vi "cRIO Main.vi"() -> ()   [LabVIEW 2015]
doc: "This application launches and executes the Tag Bus Data framework configuration for the specified target alias. This is a simple example of the framework API functions, but may also be a suitable starting point for a Host UI or Thick Client that is running a local version of the framework."
uses:
  <vilib>/NI/Module Execution Interface/Engine Runtime/Execution States.ctl
  <vilib>/NI/Module Execution Interface/Engine Runtime/Fault.ctl
  <vilib>/NI/Tag Bus Module Framework/runtime/error classification.ctl
  <vilib>/Utility/RT CPU Load.ctl
  <vilib>/NI/Current Value Table/DataTypes/Double_Read.vi
  <vilib>/NI/Current Value Table/DataTypes/U64_Read.vi
  <vilib>/NI/Current Value Table/DataTypes/U32_Read.vi
  <vilib>/NI/Current Value Table/DataTypes/Boolean_Read.vi
  <vilib>/NI/Current Value Table/Type to Enum.vi
  <vilib>/NI/Current Value Table/DataTypes/Double_Type To Enum.vi
  <vilib>/NI/Current Value Table/DataTypes/U64_Type To Enum.vi
  <vilib>/NI/Current Value Table/DataTypes/U32_Type To Enum.vi
  <vilib>/NI/Current Value Table/DataTypes/Boolean_Type To Enum.vi
  <vilib>/NI/Current Value Table/FGVs/CVT Globals.vi
  <vilib>/NI/Current Value Table/FGVs/Tag Memory.vi
  <vilib>/NI/Current Value Table/Memory Block.vi
  <vilib>/NI/Current Value Table/DataTypes/Boolean_Memory Block.vi
  <vilib>/NI/Current Value Table/DataTypes/U32_Memory Block.vi
  <vilib>/NI/Current Value Table/DataTypes/U64_Memory Block.vi
  <vilib>/NI/Current Value Table/DataTypes/Double_Memory Block.vi
  <vilib>/NI/Module Execution Interface/Engine Runtime/Engine Runtime Interface.lvclass
  <vilib>/NI/DCAF/Tag Editor Core/Framework Configuration Classes/target runtime/PL_Target Runtime.lvclass
  <vilib>/NI/Tag Bus Module Framework/runtime/TBM module execution interface.lvclass
  <vilib>/NI/Current Value Table/Current Value Table.lvlib
  <vilib>/NI_Real-Time Target Support.lvlib
panel:
  out "CPU loads":T1[](array[typedef]) {"ISR (%)" format="%#.2f"; "Idle (%)" format="%#.2f"; "Background (%)" format="%#.2f"; "Normal (%)" format="%#.2f"; "Above Normal (%)" format="%#.2f"; "High (%)" format="%#.2g"; "Timed Structures (%)" format="%#.2g"; "Time Critical (%)" format="%#.2g"; "Total (%)" format="%#.2g"}
  out "Time Structures":dbl
  out "Total":dbl
  in  "stop 2":bool
  out "error out 2":errorcluster
  out "Exec Time":u64
  out "Iterate DT":u64
  out "Late Count":u32
  out "Late":bool
  out "error out":errorcluster
  out "Duration Outputs":dbl
  out "Duration Process":dbl
  out "Duration Inputs":dbl
  out "Iter Start Time":dbl
  in  "configuration file path":path=path "/home/lvuser/benchmark_scan_IO_2x9205.pcfg"
  in  "target alias":string="dcaf_9068"
  out "engine status":T5(array[cluster])
  in  "stop":bool
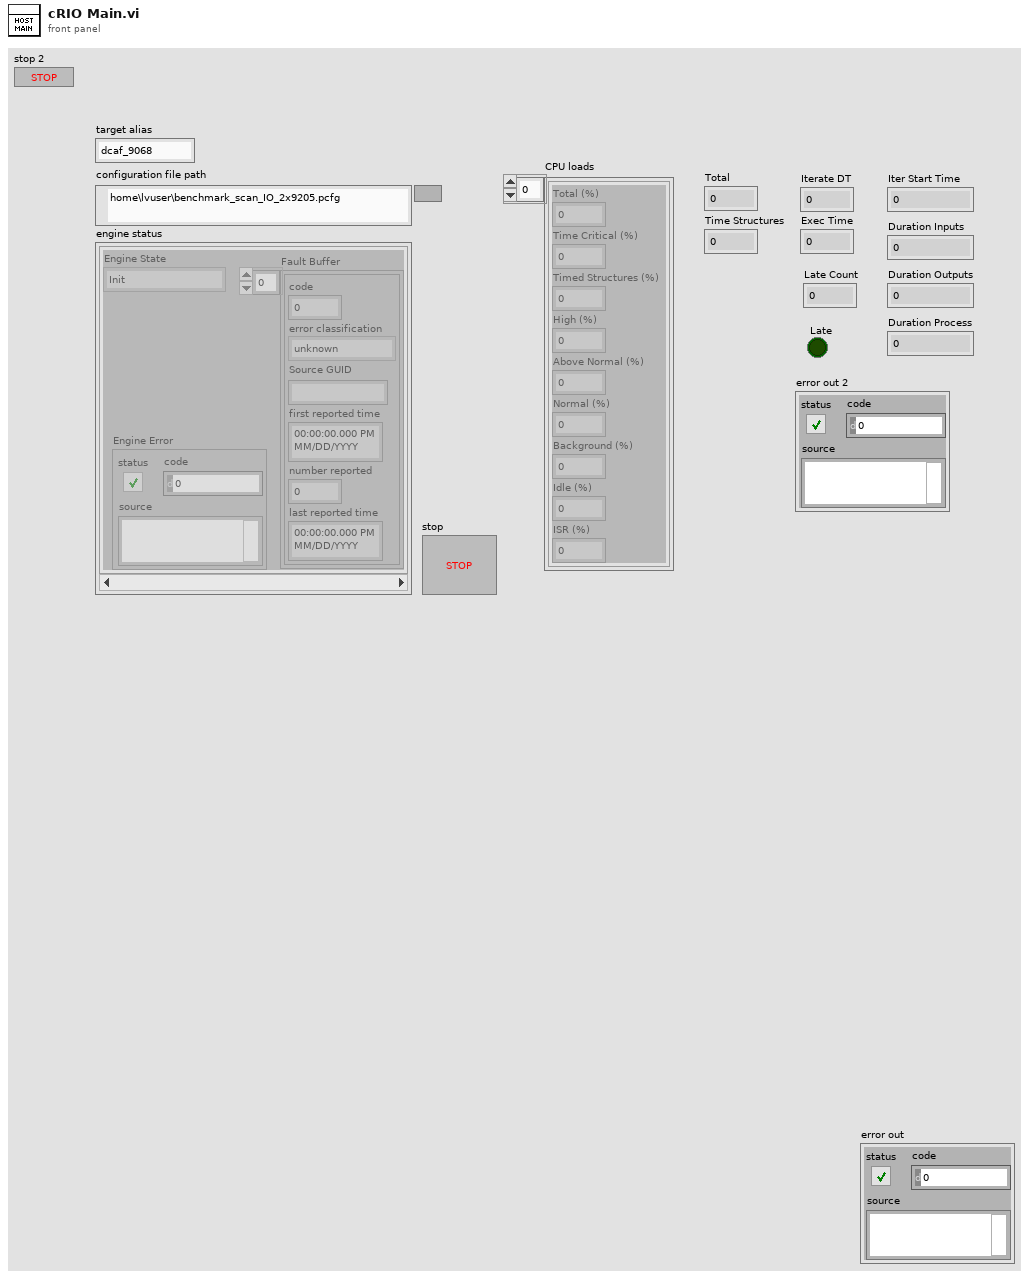
[diagram p1: front panel]
types:
  T1 = typedef "NI_Real-Time Target Support.lvlib/RT CPU Load.ctl" = cluster{"Total (%)":dbl, "Time Critical (%)":dbl, "Timed Structures (%)":dbl, "High (%)":dbl, "Above Normal (%)":dbl, "Normal (%)":dbl, "Background (%)":dbl, "Idle (%)":dbl, "ISR (%)":dbl}
  T2 = typedef "Engine Runtime Interface.lvclass/Execution States.ctl" = enum16{"Init", "Pre-Operational", "Safe-Operational", "Operational", "Stopped"}
  T3 = typedef "Engine Runtime Interface.lvclass/Fault.ctl" = cluster{"code":i32, "error classification":T4, "Source GUID":string, "first reported time":timestamp, "number reported":u32, "last reported time":timestamp}
  T4 = typedef "TBM module execution interface.lvclass/error classification.ctl" = enum16{"unknown", "none", "trivial", "recoverable", "critical"}
  T5 = cluster{"Engine State":T2, "Fault Buffer":T3[], "Engine Error":errorcluster}[]
  T6 = cluster{"Engine State":T2, "Fault Buffer":T3[], "Engine Error":errorcluster}
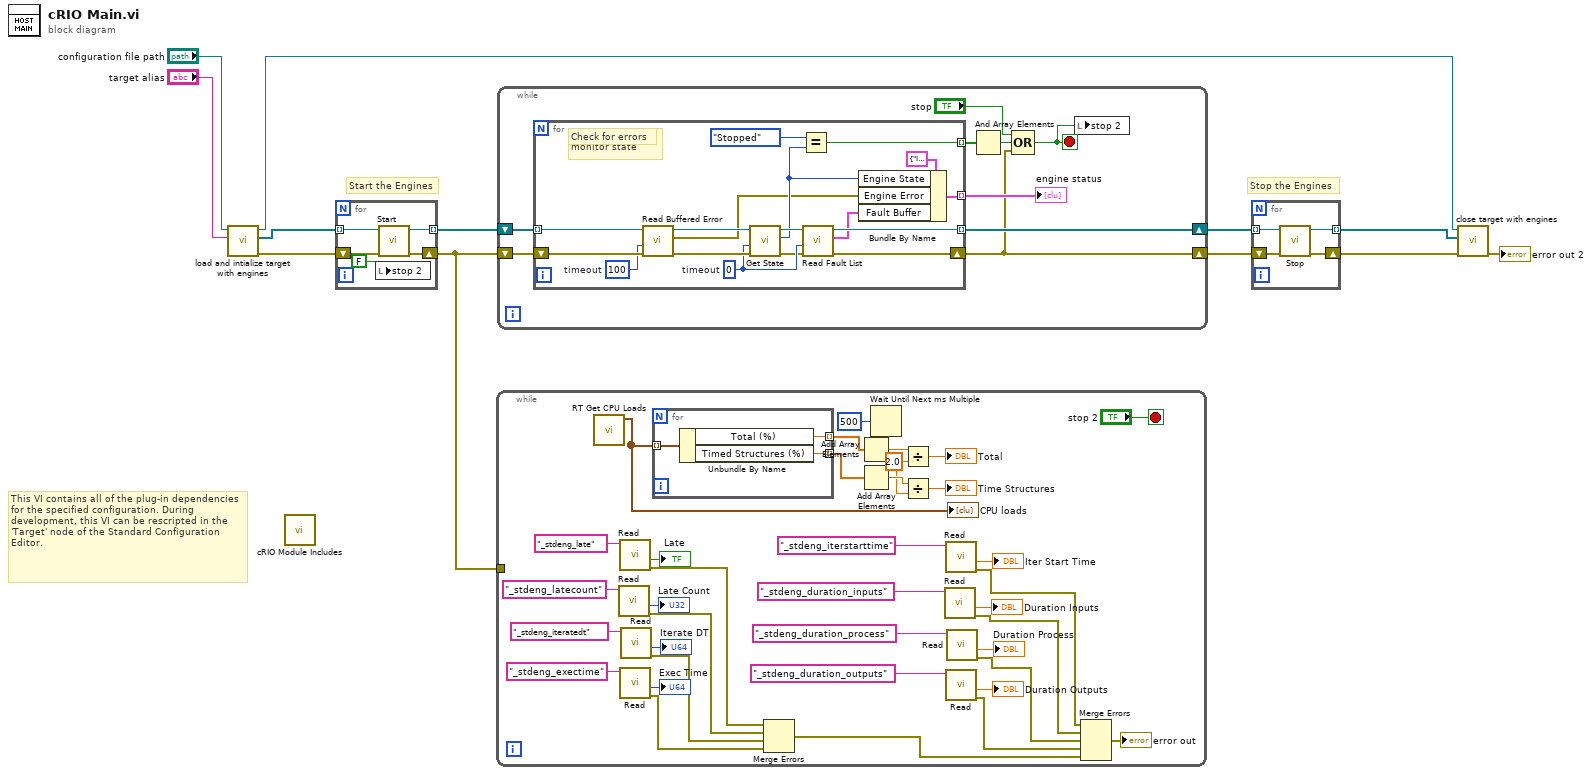
[diagram p0: block diagram]
diagram:
  # "Start the Engines"
  # "Stop the Engines"
  # "This VI contains all of the plug-in dependencies for the specified configuration. During development, this VI can be rescripted in the 'Target' node of the Standard Configuration Editor."
  n1 = call <vilib>:"load and intialize target with engines.vi"("target alias"="target alias", "file path"="configuration file path") -> ("error out"=w9:errorcluster, "engine runtime interfaces"=w8:refnum<class "Engine Runtime Interface.lvclass">[], "target runtime"=w5:refnum<class "PL_Target Runtime.lvclass">)  [unwired: 7 in]
  n2 = call "cRIO Module Includes.vi"() -> ()  [unwired: 12 in]
  n3 = for {
    tunnel: [w17] -> w12 mode=indexing
    tunnel: w8 -> [w14] mode=indexing
    shift-right: [w16] -> w1
    shift-left: w9 -> [w15]
    n4 = local write "stop 2"(FALSE ("stop 2")) -> ()
    n5 = call-dynamic "Start.vi"("error in"=w15, "Engine Runtime Interface in"=w14) -> ("error out"=w16:errorcluster, "Engine Runtime Interface out"=w17:refnum<class "Engine Runtime Interface.lvclass">)  [unwired: 8 in]
  }
  n6 = while {
    tunnel: w1 -> [_]
    stop <- "stop 2" stop-if-true
    w20 = 2.0 ("y")
    n7 = call <vilib>:"RT Get CPU Loads.vi"() -> ("CPU loads"=w25:T1[])  [unwired: 10 in, 1 out]
    "CPU loads" <- w25
    n8 = call-poly <vilib>:"Read.vi"("Tag Name"="_stdeng_latecount") -> ("error out"=w43:errorcluster, "Value"=→"Late Count":u32)  [unwired: 9 in]
    n9 = call-poly <vilib>:"Read.vi"("Tag Name"="_stdeng_late") -> ("error out"=w42:errorcluster, "Value"=→"Late":bool)  [unwired: 9 in]
    n10 = call-poly <vilib>:"Read.vi"("Tag Name"="_stdeng_exectime") -> ("error out"=w45:errorcluster, "Value"=→"Exec Time":u64)  [unwired: 9 in]
    n11 = call-poly <vilib>:"Read.vi"("Tag Name"="_stdeng_iteratedt") -> ("error out"=w44:errorcluster, "Value"=→"Iterate DT":u64)  [unwired: 9 in]
    n12 = for {
      tunnel: w25 -> [w56] mode=indexing
      tunnel: [w55] -> w24 mode=indexing
      tunnel: [w54] -> w23 mode=indexing
      n13 = Unbundle By Name(w56) -> ("Total (%)"=w55:dbl, "Timed Structures (%)"=w54:dbl)
    }
    n14 = Merge Errors(w42, w43, w44, w45) -> (w46:errorcluster)
    n15 = Add Array Elements(numeric array=w24) -> (sum=w22:dbl)
    n16 = Add Array Elements(numeric array=w23) -> (sum=w21:dbl)
    n17 = Wait Until Next ms Multiple(millisecond multiple=u32 500) -> ()  [unwired: 1 out]
    n18 = Divide(x=w22, y=w20) -> (x/y=→"Total":dbl)
    n19 = Divide(x=w21, y=w20) -> (x/y=→"Time Structures":dbl)
    n20 = call-poly <vilib>:"Read.vi"("Tag Name"="_stdeng_duration_inputs") -> ("error out"=w39:errorcluster, "Value"=→"Duration Inputs":dbl)  [unwired: 9 in]
    n21 = call-poly <vilib>:"Read.vi"("Tag Name"="_stdeng_iterstarttime") -> ("error out"=w38:errorcluster, "Value"=→"Iter Start Time":dbl)  [unwired: 9 in]
    n22 = call-poly <vilib>:"Read.vi"("Tag Name"="_stdeng_duration_outputs") -> ("error out"=w41:errorcluster, "Value"=→"Duration Outputs":dbl)  [unwired: 9 in]
    n23 = call-poly <vilib>:"Read.vi"("Tag Name"="_stdeng_duration_process") -> ("error out"=w40:errorcluster, "Value"=→"Duration Process":dbl)  [unwired: 9 in]
    n24 = Merge Errors(w38, w39, w40, w41, w46) -> (→"error out":errorcluster)
  }
  n25 = while {
    shift-right: [w63] -> w11
    shift-left: w12 -> [w65]
    shift-right: [w58] -> w10
    shift-left: w1 -> [w64]
    stop <- w57 stop-if-true
    n26 = for {
      tunnel: w65 -> [w82] mode=indexing
      tunnel: [w74] -> w63 mode=indexing
      tunnel: [w77] -> w60 mode=indexing
      shift-right: [w73] -> w58
      shift-left: w64 -> [w81]
      tunnel: [w69] -> w61 mode=indexing
      w72 = 0  # timeout
      w76 = 100  # timeout
      # "For each engine, \nmonitor state"
      # "Check for errors"
      n27 = call-dynamic "Read Buffered Error.vi"("error in"=w81, "timeout in ms (0)"=w76, "Engine Runtime Interface in"=w82) -> ("error out"=w79:errorcluster, "Engine Error"=w67:errorcluster, "Engine Runtime Interface out"=w80:refnum<class "Engine Runtime Interface.lvclass">)  [unwired: 6 in]
      n28 = call-dynamic "Get State.vi"("error in"=w79, "timeout (-1)"=w72, "Engine Runtime Interface in"=w80) -> ("error out"=w66:errorcluster, "Engine State"=w71:T2, "Engine Runtime Interface out"=w75:refnum<class "Engine Runtime Interface.lvclass">)  [unwired: 6 in]
      n29 = Equal?(x=Execution_States."Stopped" ("Engine State"), y=w71) -> (x = y?=w77:bool)
      n30 = call-dynamic "Read Fault List.vi"("error in"=w66, "timeout (-1)"=w72, "Engine Runtime Interface in"=w75) -> ("error out"=w73:errorcluster, "faults"=w70:T3[], "Engine Runtime Interface out"=w74:refnum<class "Engine Runtime Interface.lvclass">)  [unwired: 6 in]
      n31 = Bundle By Name(cluster=T6 {"Engine State"=enum."Init", "Fault Buffer"=[], "Engine Error"={"status"=FALSE, "code"=0, "source"=""}}, "Engine State"=w71, "Engine Error"=w67, "Fault Buffer"=w70) -> (w69:T6)
    }
    "engine status" <- w61
    n32 = And Array Elements(Boolean array=w60) -> (logical AND=w59:bool)
    n33 = Compound Arithmetic op=OR("stop", w59, w58) -> (w57:bool)
    n34 = local write "stop 2"(w57) -> ()
  }
  n35 = for {
    tunnel: w11 -> [w86] mode=indexing
    shift-right: [w83] -> w4
    shift-left: w10 -> [w85]
    tunnel: [w84] -> w6 mode=indexing
    n36 = call-dynamic "Stop.vi"("error in"=w85, "Engine Runtime Interface in"=w86) -> ("error out"=w83:errorcluster, "Engine Runtime Interface out"=w84:refnum<class "Engine Runtime Interface.lvclass">)  [unwired: 8 in]
  }
  n37 = call <vilib>:"close target with engines.vi"("error in"=w4, "Engine Runtime Interfaces"=w6, "Target Runtime"=w5) -> ("error out"=→"error out 2":errorcluster)  [unwired: 8 in]
